vi "RT AO FGV.vi"(7 "Enum":T1, 9 "Start Time":timestamp, 10 "AO Channel Names":string[](array[string]), 11 "AO in":dbl[](array[numeric])) -> (1 "AO Waveform":waveform(dbl)[](array[waveform]), 2 "AO  Names out":string[](array[string]), 3 "AO out":dbl[](array[numeric]))   [LabVIEW 2022 SP3]
uses:
  RT Controls/AO FGV.ctl
panel:
  out "x-y":dbl
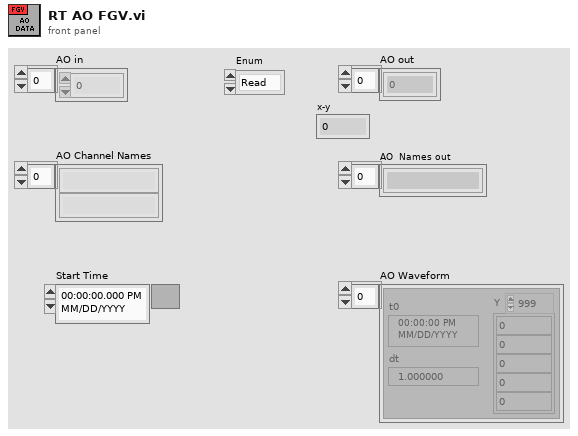
[diagram p1: front panel]
types:
  T1 = typedef "AO FGV.ctl" = enum16{"Read", "Write", "Start time", "init", "Read Only"}
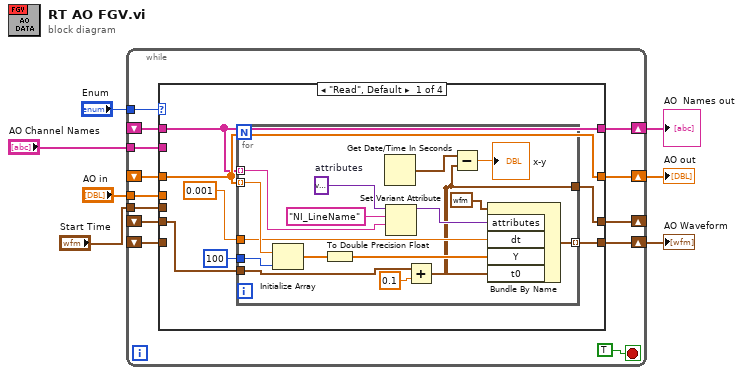
[diagram p0: block diagram]
diagram:
  n1 = while {
    tunnel: "Enum" -> [w19]
    tunnel: "AO in" -> [w18]
    shift-right: [w17] -> w4
    shift-left: _ -> [w16]
    tunnel: "Start Time" -> [w15]
    shift-right: [w14] -> _
    shift-left: _ -> [w13]
    shift-right: [w8] -> w5
    shift-left: _ -> [w12]
    shift-right: [w10] -> w1
    shift-left: _ -> [w11]
    tunnel: "AO Channel Names" -> [w9]
    stop <- TRUE stop-if-true
    n2 = case shown="\"Read\", Default" w19 {
      tunnel: w18 -> [_ _ w51 _]
      tunnel: [w25 w47 w51 w53] -> w17
      tunnel: w16 -> [w25 w47 _ w53]
      tunnel: w15 -> [_ _ _ w55]
      tunnel: [w23 w46 w50 w55] -> w14
      tunnel: w13 -> [w22 w46 w50 _]
      tunnel: [w26 w44 w49 w54] -> w8
      tunnel: w12 -> [_ w44 w49 w54]
      tunnel: w11 -> [w24 w45 w48 _]
      tunnel: [w24 w45 w48 w52] -> w10
      tunnel: w9 -> [_ _ _ w52]
      frame "Read", Default {
        n3 = for {
          tunnel: w25 -> [w42] mode=indexing
          tunnel: [w43] -> w26 mode=indexing
          tunnel: 100 ("Size") -> [w39]
          tunnel: w24 -> [w37] mode=indexing
          tunnel: 0.001 ("dt(sec)") -> [w34]
          tunnel: [w29] -> w23
          tunnel: w22 -> [w32]
          w38 = variant  # attributes
          n4 = Initialize Array(w42, w39) -> (w41:dbl[])
          n5 = To Double Precision Float(number=w41) -> (double precision float=w40:dbl[])
          n6 = Get Date/Time In Seconds() -> (seconds since 1Jan1904=w30:timestamp)
          n7 = Set Variant Attribute(Variant=w38, name="NI_LineName", value=w37) -> (Variant out=w33:variant)  [unwired: 1 in, 2 out]
          n8 = Add(x=w32, y=0.1) -> (x+y=w29:timestamp)
          n9 = Subtract(x=w30, y=w29) -> (x-y=→"x-y":dbl)
          n10 = Bundle By Name(cluster=waveform(dbl) {"t0"=timestamp(0 s since 1904-01-01), "dt"=1.0, "Y"=[]} ("waveform"), "attributes"=w33, "dt"=w34, "Y"=w40, "t0"=w29) -> (w43:waveform(dbl))
        }
      }
      frame "Read Only" {
      }
      frame "Write" {
      }
      frame "Start time" {
      }
    }
  }
  "AO Waveform" <- w5
  "AO out" <- w4
  "AO  Names out" <- w1
